vi "imp_test_v7.vi"() -> ()   [LabVIEW 2014]
uses:
  <vilib>/LabVIEW Targets/FPGA/cRIO/shared/nicrio_ModuleControls/nicrio_cRIO-9237_DataRatesRing.ctl
  <vilib>/LabVIEW Targets/FPGA/cRIO/shared/nicrio_ModuleControls/nicrio_cRIO-9237_ExcitationVoltageRing.ctl
  <vilib>/rvi/FXPMathLib/FxpSinAndCos/subVIs/nifxpmath_SinAndCos_SimConfig.ctl
  <vilib>/rvi/Emulation/niFpgaGetClockAttributes.vi
  <vilib>/rvi/Emulation/niFpgaSctlEmulationGetInTimedLoop.vi
  <vilib>/rvi/Emulation/niFpgaEmulationReportErrorSimple.vi
  <vilib>/rvi/Emulation/niFpgaProcessEmulError.vi
  <vilib>/rvi/interface/RandomDataEmulation/nirviRandomDataMultiElementFPGAFIFO.vi
  <instcachedir>/0/nirviRandomDataMultiElementFPGAFIFO_AD0CFC12EF974623A9C2E4184BC062B2.lvgen/nirviRandomDataMultiElementFPGAFIFO_AD0CFC12EF974623A9C2E4184BC062B2_025.vi
  <vilib>/rvi/interface/RandomDataEmulation/niFpgaRandomDataHandleErrors.vi
  <vilib>/rvi/Emulation/niFpgaCriticalErrorInLSC.vi
  <vilib>/rvi/eio/common/nirviEmuTemplateMethod_errors.vi
  <vilib>/rvi/FXPMathLib/FxpSinAndCos/simVIs/DllFxpSinAndCosTemp_sub.vi
  <vilib>/rvi/eio/common/nirviEmuTemplatePropertySet_errors.vi
  <vilib>/rvi/DataTransferAndStorage/Container/XNode/niFpgaContainer.xnode
  <vilib>/rvi/interface/RandomDataEmulation/nirviRandomDataFpgaMultiElementTemplate.vi
  <vilib>/eio/EIONode/EIONode.xnode
  <vilib>/rvi/FXPMathLib/FxpMul/XNode/nifxpmath_Multiplier.xnode
  <vilib>/rvi/FXPMathLib/FxpSinAndCos/XNode/nifxpmath_SinAndCos.xnode
  <vilib>/rvi/Analysis/measure/butterworth/XNode/niFpgaButterworthFilter.xnode
  <vilib>/rvi/FXPMathLib/FxpSub/XNode/nifxpmath_Sub.xnode
  <vilib>/rvi/FXPMathLib/FxpAdd/XNode/nifxpmath_Add.xnode
  <vilib>/eio/EIOPropertyNode/EIOPropertyNode.xnode
  <vilib>/rvi/eio/common/nirviEmuTemplatePropertyGet_errors.vi
  <vilib>/rvi/eio/common/nirviEmuTemplatePropertyGet_noerrors.vi
  <vilib>/rvi/eio/common/nirviEmuTemplatePropertySet_noerrors.vi
  <vilib>/rvi/FXPMathLib/sim/FxpSim.dll
panel:
  in  "Belt_op":fxp<+/-,7,7>
  in  "Belt_mp":fxp<+/-,6,6>
  in  "Belt_oy":fxp<+/-,7,7>
  in  "Belt_my":fxp<+/-,6,6>
  out "Fp_dc":fxp<+/-,32,10>
  out "Fy_dc":fxp<+/-,32,10>
  in  "Zero_y":bool
  in  "Zero_p":bool
  in  "mt0_omega_p":u32
  in  "Encoder reset":bool
  out "fpt_d":fxp<+/-,36,18>
  out "Dp_error_dd":fxp<+/-,36,16>
  out "Dp_error_d":fxp<+/-,33,8>
  in  "Dp_dd coeff.":i32[](array[numeric])=[946630756, 63555534]
  out "Dp_dd":fxp<+/-,36,25>
  out "dFp_PID":fxp<+/-,36,18>
  in  "dFp_PID coeff.":i32[](array[numeric])=[946630756, 63555534]
  out "fpt_i":fxp<+/-,34,18>
  in  "Bv_p":fxp<+/-,22,8>
  in  "Kv_p":fxp<+/-,22,8>
  out "Dp_error":fxp<+/-,22,7>
  out "Dpr_sin":fxp<+/-,22,7>
  in  "Sin offset_p":fxp<+/-,22,7>
  in  "Sin magnitude_p":fxp<+/-,21,6>
  out "Dpr_sin_dd":fxp<+/-,35,20>
  out "Dpr_sin_d":fxp<+/-,33,15>
  out "Sin omega_p":fxp<+/-,34,9>
  in  "Sin wave freq._p (Hz)":fxp<+/-,32,6>
  in  "Dpr_step":fxp<+/-,22,7>
  out "Dpr_for":fxp<+/-,22,7>
  in  "Command_p":i16(ring) items=["Step", "Sine"]
  in  "Ki_p":fxp<+/-,36,9>
  out "Fp_PID":fxp<+/-,36,16>
  in  "fp_tolorance":fxp<+,22,6>
  out "fp_tilde":fxp<+/-,33,10>
  in  "Kd_p":fxp<+/-,36,9>
  in  "Kp_p":fxp<+/-,36,9>
  out "Fr_p":fxp<+/-,32,10>
  in  "S/F coeff_p":fxp<+/-,25,-10>
  in  "S/F coeff_y":fxp<+/-,25,-10>
  out "va_p":fxp<+/-,36,7>
  out "vb_p":fxp<+/-,37,8>
  out "vq_p_F":fxp<+/-,20,5> format="%.57g"
  out "vd_p_F":fxp<+/-,20,5>
  in  "dFp_add":bool
  in  "Stop motor_p":bool
  out "Force_p":fxp<+/-,32,10>
  in  "Strain selection_p":i16(ring) items=["Raw", "Avg.8", "Avg.8 w. filter"]
  out "Strain_p (Avg8 w. f)":fxp<+/-,36,8>
  in  "Strain_p Avg.8 coeff.":i32[](array[numeric])=[946630756, 63555534]
  out "Strain_p (Avg8)":fxp<+/-,36,4>
  out "Raw Strain_p":fxp<+/-,36,4>
  out "Mod6/AI3":fxp<+/-,36,4>
  in  "Strain gage reset_p":bool
  out "Dp_d (mm/s)":fxp<+/-,36,11>
  out "omega_p (rad/s)":fxp<+/-,20,9>
  out "mt_omega_p":u32
  out "rad_p(NrTheta)":fxp<+/-,33,20>
  out "D_p(mm)":fxp<+/-,32,7>
  out "Encoder Position_p":i32
  in  "Encoder reset_p":bool
  out "Strain_y (Avg8 w. f)":fxp<+/-,36,8>
  in  "Strain_y Avg8 coeff.":i32[](array[numeric])=[-898916953, 1957103773, 3888751]
  out "Dyr_for":fxp<+/-,22,7>
  in  "Command_y":i16(ring) items=["Step", "Sine"]
  out "Strain_y (Avg8)":fxp<+/-,36,4>
  in  "Strain selection_y":i16(ring) items=["Raw", "Avg.8", "Avg.8 w. filter"]
  out "vb_y":fxp<+/-,38,8>
  out "va_y":fxp<+/-,38,8>
  out "fyt_d":fxp<+/-,36,18>
  out "Fr_y":fxp<+/-,32,10>
  in  "Bv_y":fxp<+/-,22,8>
  out "Dy_error_dd":fxp<+/-,36,16>
  out "Dy_error_d":fxp<+/-,33,8>
  in  "Kv_y":fxp<+/-,22,8>
  out "Dy_error":fxp<+/-,22,7>
  out "Dyr_sin_dd":fxp<+/-,35,20>
  out "Dyr_sin_d":fxp<+/-,33,15>
  out "Sin omega_y":fxp<+/-,34,9>
  out "Dyr_sin":fxp<+/-,22,7>
  in  "Sin offset_y":fxp<+/-,22,7>
  in  "Sin magnitude_y":fxp<+/-,21,6>
  out "Time now(s)":fxp<+,52,14>
  in  "Sin wave freq._y (Hz)":fxp<+/-,32,6>
  in  "Dyr_step":fxp<+/-,22,7>
  in  "Drive mode":i16(ring) items=["Backward", "Forward"]
  out "Dy_dd":fxp<+/-,36,25>
  in  "Dy_dd coeff.":i32[](array[numeric])=[946630756, 63555534]
  out "dFy_PID":fxp<+/-,36,18>
  in  "dFy_PID coeff.":i32[](array[numeric])=[946630756, 63555534]
  out "fyt_i":fxp<+/-,36,16>
  out "Fy_PID":fxp<+/-,36,16>
  in  "fy_tolorance":fxp<+,22,6>
  in  "Ki_y":fxp<+/-,36,9>
  in  "Kd_y":fxp<+/-,36,9>
  out "fy_tilde":fxp<+/-,32,10>
  in  "Kp_y":fxp<+/-,36,9>
  out "vq_y_F":fxp<+/-,20,5> format="%.57g"
  out "vd_y_F":fxp<+/-,20,5>
  in  "dFy_add":bool
  in  "Stop motor_y":bool
  out "Dy_d (mm/s)":fxp<+/-,36,11>
  out "omega_y (rad/s)":fxp<+/-,20,9>
  in  "mt0_omega_y":u32
  out "mt_omega_y":u32
  out "rad_y(NrTheta)":fxp<+/-,33,20>
  out "D_y(mm)":fxp<+/-,32,7>
  out "Encoder Position_y":i32
  in  "Encoder reset_y":bool
  in  "Ini coe.":bool
  out "Loop rate (kHz)":fxp<+/-,36,7>
  out "Force_y":fxp<+/-,32,10>
  out "Raw Strain_y":fxp<+/-,36,4>
  in  "Strain gage reset_y":bool
  in  "Stop (Strain)":bool
  out "Mod6/AI2":fxp<+/-,36,4>
  in  "Excitation Voltage":T1 items=["2.5 Volts", "3.3 Volts", "5.0 Volts", "10.0 Volts", "External Excitation"]
  in  "Data Rate":T2=1 items=["50.000 kS/s (NI 9237)"=1, "25.000 kS/s (NI 9237)"=2, "16.667 kS/s (NI 9237)"=3, "12.500 kS/s (NI 9237)"=4, "10.000 kS/s (NI 9237)"=5, "8.333 kS/s (NI 9237)"=6, "7.143 kS/s (NI 9237)"=7, "6.250 kS/s (NI 9237)"=8, "5.556 kS/s (NI 9237)"=9, "5.000 kS/s (NI 9237)"=10, "4.545 kS/s (NI 9237)"=11, "4.167 kS/s (NI 9237)"=12, "3.846 kS/s (NI 9237)"=13, "3.571 kS/s (NI 9237)"=14, "3.333 kS/s (NI 9237)"=15, "3.125 kS/s (NI 9237)"=16, "2.941 kS/s (NI 9237)"=17, "2.778 kS/s (NI 9237)"=18, "2.632 kS/s (NI 9237)"=19, "2.500 kS/s (NI 9237)"=20, "2.381 kS/s (NI 9237)"=21, "2.273 kS/s (NI 9237)"=22, "2.174 kS/s (NI 9237)"=23, "2.083 kS/s (NI 9237)"=24, "2.000 kS/s (NI 9237)"=25, "1.923 kS/s (NI 9237)"=26, "1.852 kS/s (NI 9237)"=27, "1.786 kS/s (NI 9237)"=28, "1.724 kS/s (NI 9237)"=29, "1.667 kS/s (NI 9237)"=30, "1.613 kS/s (NI 9237)"=31]
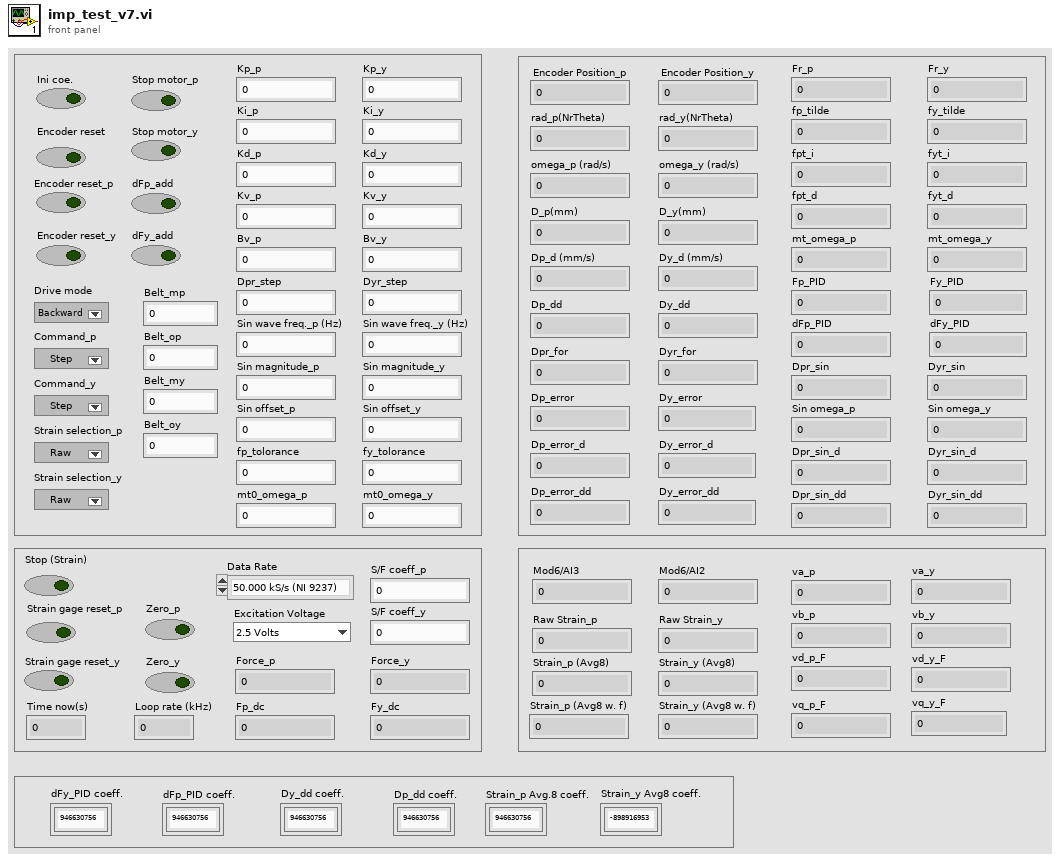
[diagram p1: front panel]
types:
  T1 = typedef "nicrio_cRIO-9237_ExcitationVoltageRing.ctl" = u8
  T2 = typedef "nicrio_cRIO-9237_DataRatesRing.ctl" = u8
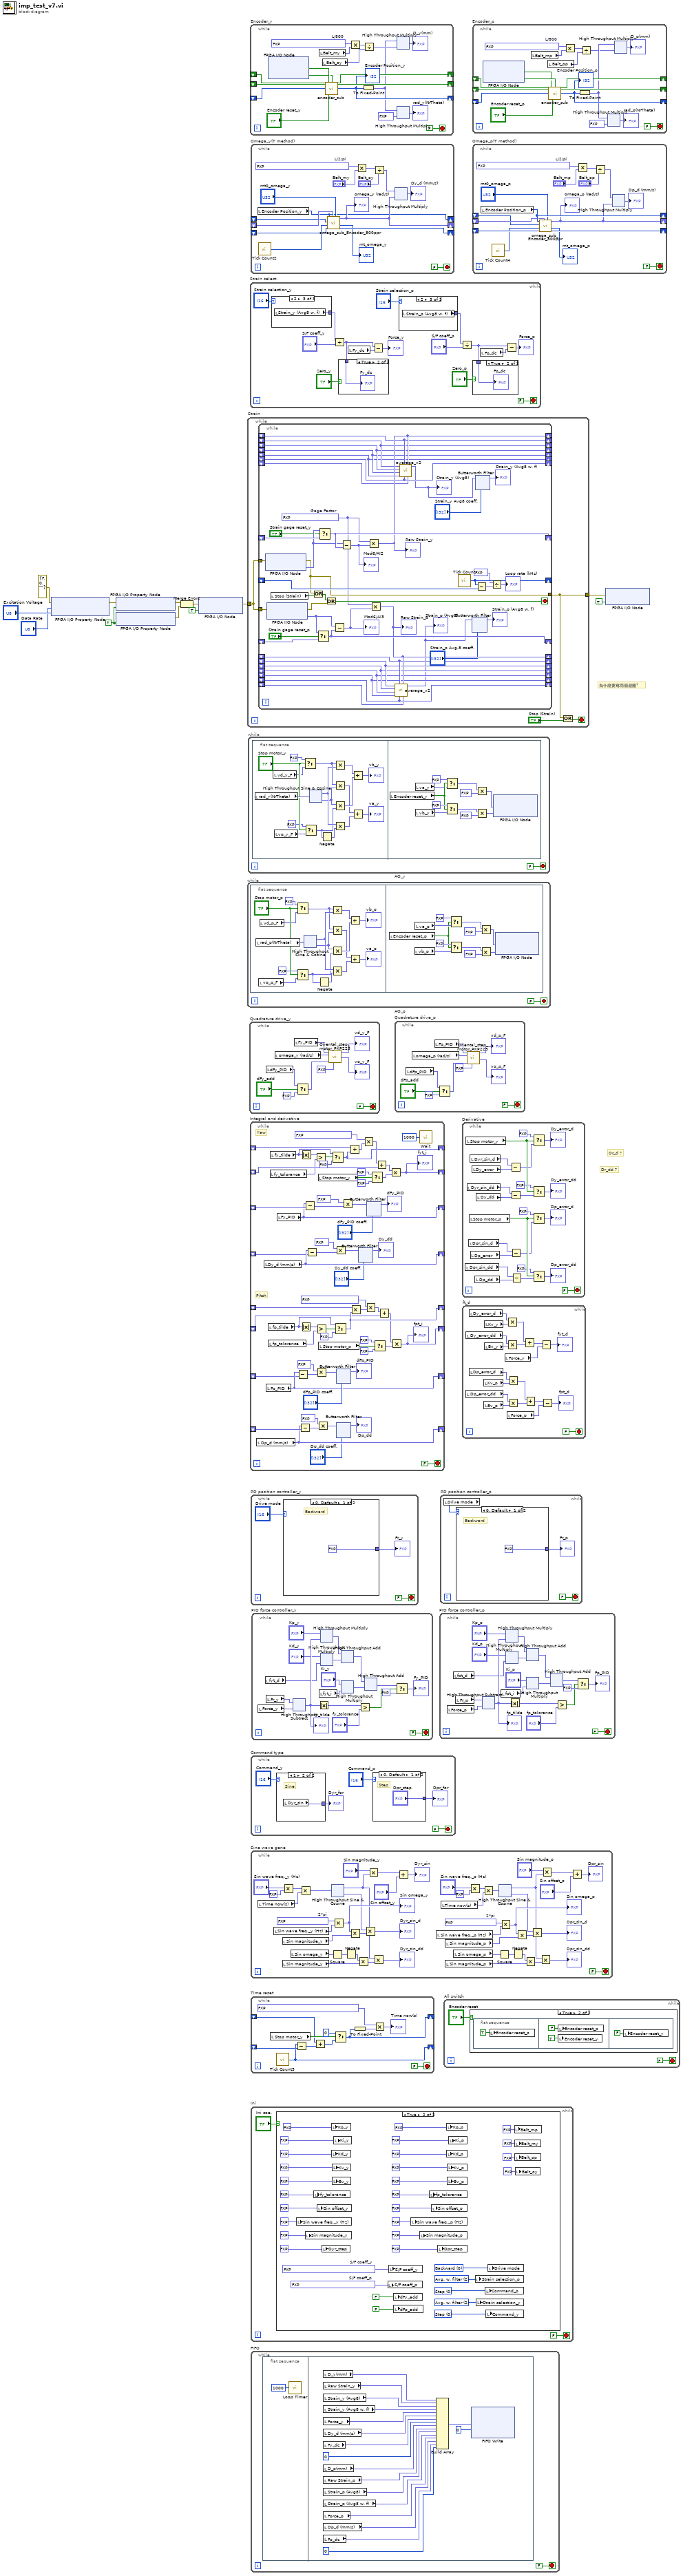
[diagram p0: block diagram]
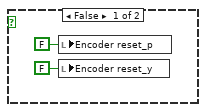
[diagram p2: hidden frame]
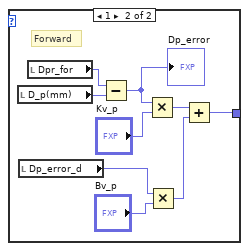
[diagram p3: hidden frame]
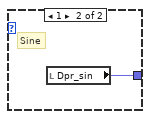
[diagram p4: hidden frame]
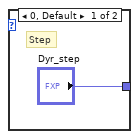
[diagram p5: hidden frame]
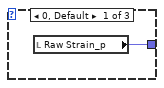
[diagram p8: hidden frame]
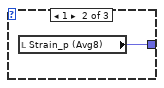
[diagram p9: hidden frame]
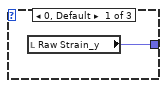
[diagram p10: hidden frame]
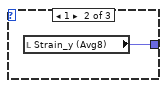
[diagram p11: hidden frame]
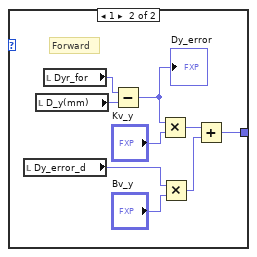
[diagram p12: hidden frame]
diagram:
  w5 = TRUE ("Half-Bridge Enable")
  # "為什麼要寫兩個迴圈?"
  # "Dr_dd ?"
  # "Dr_d ?"
  n1 = xnode "FPGA I/O Property Node"("error in"=errorcluster {"status"=FALSE, "code"=0, "source"=""}, "Data Rate"="Data Rate", "Excitation Voltage"="Excitation Voltage") -> ("error out"=w10:errorcluster)  [unwired: 1 in, 1 out]
  n2 = xnode "FPGA I/O Property Node"("error in"=w10, "Half-Bridge Enable"=w5) -> ("error out"=w3:errorcluster)  [unwired: 1 in, 1 out]
  n3 = xnode "FPGA I/O Property Node"("Half-Bridge Enable"=w5) -> ("error out"=w2:errorcluster)  [unwired: 2 in, 1 out]
  n4 = Merge Errors(w3, w2) -> (w4:errorcluster)
  n5 = xnode "FPGA I/O Node"("error in"=w4, "Mod6/Start"=TRUE) -> ("error out"=w8:errorcluster)  [unwired: 1 in, 1 out]
  n6 = while "Strain" {
    tunnel: w8 -> [w15]
    tunnel: [w13] -> w1
    stop <- w14 stop-if-true
    n7 = while {
      tunnel: w15 -> [w61]
      tunnel: [w34] -> w13
      shift-right: [w58] -> _
      shift-left: _ -> [w59]
      shift-right: [w54] -> _
      shift-left: _ -> [w55]
      shift-right: [w49] -> _
      shift-left: _ -> [w48]
      shift-right: [w48] -> _
      shift-left: _ -> [w47]
      shift-right: [w47] -> _
      shift-left: _ -> [w46]
      shift-right: [w46] -> _
      shift-left: _ -> [w45]
      shift-right: [w45] -> _
      shift-left: _ -> [w44]
      shift-right: [w44] -> _
      shift-left: _ -> [w43]
      shift-right: [w43] -> _
      shift-left: _ -> [w42]
      tunnel: w15 -> [w38]
      shift-right: [w31] -> _
      shift-left: _ -> [w32]
      shift-right: [w27] -> _
      shift-left: _ -> [w26]
      shift-right: [w26] -> _
      shift-left: _ -> [w25]
      shift-right: [w25] -> _
      shift-left: _ -> [w24]
      shift-right: [w24] -> _
      shift-left: _ -> [w23]
      shift-right: [w23] -> _
      shift-left: _ -> [w22]
      shift-right: [w22] -> _
      shift-left: _ -> [w21]
      shift-right: [w21] -> _
      shift-left: _ -> [w20]
      stop <- w35 stop-if-true
      w29 = fxp<+,20,2> 2.115001678466797  # Gage Factor
      n8 = xnode "FPGA I/O Node"("error in"=w61) -> ("error out"=w34:errorcluster, "Mod6/AI2"=w56:fxp<+/-,24,-4>)  [unwired: 1 in, 1 out]
      n9 = xnode "FPGA I/O Node"("error in"=w38) -> ("error out"=w36:errorcluster, "Mod6/AI3"=w30:fxp<+/-,24,-4>)  [unwired: 1 in, 1 out]
      n10 = local read "Stop (Strain)"() -> (w60:bool)
      n11 = Or(x=w34, y=w60) -> (x .or. y?=w37:bool)
      n12 = Select(t=w30, s="Strain gage reset_p", f=w32) -> (s? t:f=w31:fxp<+/-,24,-4>)
      n13 = Select(t=w56, s="Strain gage reset_y", f=w59) -> (s? t:f=w58:fxp<+/-,24,-4>)
      n14 = Or(x=w37, y=w36) -> (x .or. y?=w35:bool)
      n15 = Subtract(x=w30, y=w31) -> (x-y=w28:fxp<+/-,30,-3>)
      "Mod6/AI3" <- w28
      n16 = Subtract(x=w56, y=w58) -> (x-y=w57:fxp<+/-,30,-3>)
      "Mod6/AI2" <- w57
      n17 = Multiply(x=w29, y=w57) -> (x*y=w49:fxp<+/-,41,6>)
      "Raw Strain_y" <- w49
      n18 = Multiply(x=w29, y=w28) -> (x*y=w27:fxp<+/-,50,-1>)
      "Raw Strain_p" <- w27
      n19 = call "average_v2.vi"("Numeric 8"=w20, "Numeric"=w27, "Numeric 7"=w21, "Numeric 2"=w26, "Numeric 6"=w22, "Numeric 5"=w23, "Numeric 4"=w24, "Numeric 3"=w25) -> ("Mean (8pt)"=w19:fxp<+/-,32,4>)  [unwired: 1 in, 2 out]
      "Strain_p (Avg8)" <- w19
      n20 = call "average_v2.vi"("Numeric 8"=w42, "Numeric"=w49, "Numeric 7"=w43, "Numeric 2"=w48, "Numeric 6"=w44, "Numeric 5"=w45, "Numeric 4"=w46, "Numeric 3"=w47) -> ("Mean (8pt)"=w41:fxp<+/-,32,4>)  [unwired: 1 in, 2 out]
      "Strain_y (Avg8)" <- w41
      n21 = call "Tick Count"() -> ("Tick Count(uSec)"=w54:u32)
      n22 = xnode "Butterworth Filter"("input data"=w19, "scaled coefficients"="Strain_p Avg.8 coeff.") -> ("output data"=→"Strain_p (Avg8 w. f)":fxp<+/-,36,8>)  [unwired: 1 in]
      n23 = xnode "Butterworth Filter"("input data"=w41, "scaled coefficients"="Strain_y Avg8 coeff.") -> ("output data"=→"Strain_y (Avg8 w. f)":fxp<+/-,32,4>)  [unwired: 1 in]
      n24 = Subtract(x=w54, y=w55) -> (x-y=w52:fxp<+/-,32,16>)
      n25 = Divide(x=fxp<+,7,10> 1000.0, y=w52) -> (x/y=→"Loop rate (kHz)":fxp<+/-,40,27>)
    }
    n26 = Or(x=w13, y="Stop (Strain)") -> (x .or. y?=w14:bool)
  }
  n27 = while "AO_p" {
    stop <- FALSE stop-if-true
    n28 = flat-sequence {
      frame #0 {
        n29 = local read "rad_p(NrTheta)"() -> (w90:fxp<+/-,33,20>)
        n30 = local read "vq_p_F"() -> (w91:fxp<+/-,20,5>)
        n31 = local read "vd_p_F"() -> (w93:fxp<+/-,20,5>)
        n32 = Select(t=fxp<+/-,20,5> 0.0, s="Stop motor_p", f=w93) -> (s? t:f=w82:fxp<+/-,20,5>)
        n33 = Select(t=fxp<+,1,1> 0.0, s="Stop motor_p", f=w91) -> (s? t:f=w81:fxp<+/-,20,5>)
        n34 = xnode "High Throughput Sine & Cosine"("x (pi)"=w90) -> ("sin(x)"=w84:fxp<+/-,16,2>, "cos(x)"=w83:fxp<+/-,16,2>)
        n35 = Negate(x=w81) -> (-x=w89:fxp<+/-,21,6>)
        n36 = Multiply(x=w82, y=w84) -> (x*y=w88:fxp<+/-,36,7>)
        n37 = Multiply(x=w82, y=w83) -> (x*y=w86:fxp<+/-,36,7>)
        n38 = Multiply(x=w83, y=w81) -> (x*y=w87:fxp<+/-,36,7>)
        n39 = Multiply(x=w84, y=w89) -> (x*y=w85:fxp<+/-,35,6>)
        n40 = Add(x=w88, y=w87) -> (x+y=→"vb_p":fxp<+/-,37,8>)
        n41 = Add(x=w86, y=w85) -> (x+y=→"va_p":fxp<+/-,36,7>)
      }
      frame #1 {
        n42 = local read "Encoder reset_p"() -> (w126:bool)
        n43 = local read "vb_p"() -> (w127:fxp<+/-,37,8>)
        n44 = local read "va_p"() -> (w128:fxp<+/-,36,7>)
        n45 = Select(t=fxp<+,2,2> 3.0, s=w126, f=w128) -> (s? t:f=w134:fxp<+/-,36,7>)
        n46 = Select(t=fxp<+,1,1> 0.0, s=w126, f=w127) -> (s? t:f=w133:fxp<+/-,37,8>)
        n47 = Multiply(x=w134, y=fxp<+/-,1,0> -0.5) -> (x*y=w129:fxp<+/-,36,6>)
        n48 = Multiply(x=w133, y=fxp<+/-,1,0> -0.5) -> (x*y=w130:fxp<+/-,36,6>)
        n49 = xnode "FPGA I/O Node"("Mod8/AO0"=w129, "Mod8/AO1"=w130) -> ()  [unwired: 2 in, 2 out]
      }
    }
  }
  n50 = while "AO_y" {
    stop <- FALSE stop-if-true
    n51 = flat-sequence {
      frame #0 {
        n52 = local read "rad_y(NrTheta)"() -> (w154:fxp<+/-,33,20>)
        n53 = local read "vd_y_F"() -> (w152:fxp<+/-,20,5>)
        n54 = local read "vq_y_F"() -> (w151:fxp<+/-,20,5>)
        n55 = Select(t=fxp<+/-,20,5> 0.0, s="Stop motor_y", f=w152) -> (s? t:f=w146:fxp<+/-,20,5>)
        n56 = Select(t=fxp<+/-,20,5> 0.0, s="Stop motor_y", f=w151) -> (s? t:f=w145:fxp<+/-,20,5>)
        n57 = xnode "High Throughput Sine & Cosine"("x (pi)"=w154) -> ("sin(x)"=w148:fxp<+/-,17,2>, "cos(x)"=w147:fxp<+/-,17,2>)
        n58 = Negate(x=w145) -> (-x=w144:fxp<+/-,21,6>)
        n59 = Multiply(x=w146, y=w148) -> (x*y=w143:fxp<+/-,37,7>)
        n60 = Multiply(x=w146, y=w147) -> (x*y=w141:fxp<+/-,37,7>)
        n61 = Multiply(x=w147, y=w145) -> (x*y=w142:fxp<+/-,37,7>)
        n62 = Multiply(x=w148, y=w144) -> (x*y=w140:fxp<+/-,36,6>)
        n63 = Add(x=w143, y=w142) -> (x+y=→"vb_y":fxp<+/-,38,8>)
        n64 = Add(x=w141, y=w140) -> (x+y=→"va_y":fxp<+/-,37,7>)
      }
      frame #1 {
        n65 = local read "Encoder reset_y"() -> (w187:bool)
        n66 = local read "va_y"() -> (w186:fxp<+/-,38,8>)
        n67 = local read "vb_y"() -> (w185:fxp<+/-,38,8>)
        n68 = Select(t=fxp<+,2,2> 3.0, s=w187, f=w186) -> (s? t:f=w191:fxp<+/-,38,8>)
        n69 = Select(t=fxp<+,1,1> 0.0, s=w187, f=w185) -> (s? t:f=w190:fxp<+/-,38,8>)
        n70 = Multiply(x=w191, y=fxp<+/-,1,0> -0.5) -> (x*y=w194:fxp<+/-,39,8>)
        n71 = Multiply(x=w190, y=fxp<+/-,1,0> -0.5) -> (x*y=w195:fxp<+/-,37,6>)
        n72 = xnode "FPGA I/O Node"("Mod8/AO2"=w194, "Mod8/AO3"=w195) -> ()  [unwired: 2 in, 2 out]
      }
    }
  }
  n73 = while "Quadrature drive_y" {
    stop <- FALSE stop-if-true
    n74 = local read "dFy_PID"() -> (w197:fxp<+/-,36,18>)
    n75 = local read "omega_y (rad/s)"() -> (w205:fxp<+/-,20,9>)
    n76 = local read "Fy_PID"() -> (w198:fxp<+/-,36,16>)
    n77 = Select(t=w197, s="dFy_add", f=fxp<+,1,1> 0.0) -> (s? t:f=w201:fxp<+/-,36,18>)
    n78 = call "Oriental_step_motor_PKP225.vi"("F_Threshold"=fxp<+,12,12> 10.0, "dFmr"=w201, "omega"=w205, "Fmr"=w198) -> ("vq_F"=→"vq_y_F":fxp<+/-,20,5>, "vd_F"=→"vd_y_F":fxp<+/-,20,5>)  [unwired: 6 in]
  }
  n79 = while "Strain select." {
    stop <- FALSE stop-if-true
    n80 = case shown="2" "Strain selection_y" {
      tunnel: [w226 w227 w228] -> w219
      frame 0, Default {
        n81 = local read "Raw Strain_y"() -> (w226:fxp<+/-,36,4>)
      }
      frame 1 {
        n82 = local read "Strain_y (Avg8)"() -> (w227:fxp<+/-,36,4>)
      }
      frame 2 {
        n83 = local read "Strain_y (Avg8 w. f)"() -> (w228:fxp<+/-,36,8>)
      }
    }
    n84 = Divide(x=w219, y="S/F coeff_y") -> (x/y=w212:fxp<+/-,32,10>)
    n85 = case shown="True" "Zero_y" {
      tunnel: w212 -> [_ w222]
      frame False {
      }
      frame True {
        "Fy_dc" <- w222
      }
    }
    n86 = local read "Fy_dc"() -> (w213:fxp<+/-,32,10>)
    n87 = Subtract(x=w212, y=w213) -> (x-y=→"Force_y":fxp<+/-,33,11>)
    n88 = case shown="2" "Strain selection_p" {
      tunnel: [w223 w224 w225] -> w217
      frame 0, Default {
        n89 = local read "Raw Strain_p"() -> (w223:fxp<+/-,36,4>)
      }
      frame 1 {
        n90 = local read "Strain_p (Avg8)"() -> (w224:fxp<+/-,36,4>)
      }
      frame 2 {
        n91 = local read "Strain_p (Avg8 w. f)"() -> (w225:fxp<+/-,36,8>)
      }
    }
    n92 = Divide(x=w217, y="S/F coeff_p") -> (x/y=w209:fxp<+/-,32,10>)
    n93 = case shown="True" "Zero_p" {
      tunnel: w209 -> [_ w221]
      frame False {
      }
      frame True {
        "Fp_dc" <- w221
      }
    }
    n94 = local read "Fp_dc"() -> (w207:fxp<+/-,32,10>)
    n95 = Subtract(x=w209, y=w207) -> (x-y=→"Force_p":fxp<+/-,33,11>)
  }
  n96 = while "Integral and derivative" {
    shift-right: [w284] -> _
    shift-left: _ -> [w283]
    shift-right: [w276] -> _
    shift-left: _ -> [w275]
    shift-right: [w286] -> _
    shift-left: _ -> [w287]
    shift-right: [w266] -> _
    shift-left: _ -> [w265]
    shift-right: [w252] -> _
    shift-left: _ -> [w255]
    shift-right: [w245] -> _
    shift-left: _ -> [w244]
    shift-right: [w239] -> _
    shift-left: _ -> [w238]
    shift-right: [w234] -> _
    shift-left: _ -> [w235]
    stop <- FALSE stop-if-true
    # "Pitch"
    # "Yaw"
    n97 = local read "Dp_d (mm/s)"() -> (w234:fxp<+/-,36,11>)
    n98 = local read "Dy_d (mm/s)"() -> (w266:fxp<+/-,36,11>)
    n99 = local read "Fp_PID"() -> (w239:fxp<+/-,36,16>)
    n100 = local read "fp_tilde"() -> (w256:fxp<+/-,33,10>)
    n101 = local read "fp_tolorance"() -> (w259:fxp<+,22,6>)
    n102 = local read "fy_tolorance"() -> (w262:fxp<+,22,6>)
    n103 = local read "fy_tilde"() -> (w288:fxp<+/-,32,10>)
    n104 = local read "Fy_PID"() -> (w286:fxp<+/-,36,16>)
    n105 = Subtract(x=w239, y=w238) -> (x-y=w243:fxp<+/-,37,17>)
    n106 = Subtract(x=w234, y=w235) -> (x-y=w236:fxp<+/-,37,12>)
    n107 = Absolute Value(x=w256) -> (abs(x)=w260:fxp<+,33,10>)
    n108 = Absolute Value(x=w288) -> (abs(x)=w290:fxp<+,32,10>)
    n109 = Subtract(x=w286, y=w287) -> (x-y=w274:fxp<+/-,37,17>)
    n110 = Subtract(x=w266, y=w265) -> (x-y=w268:fxp<+/-,36,11>)
    n111 = Greater?(x=w290, y=w262) -> (0:w291:bool)
    n112 = Greater?(x=w260, y=w259) -> (0:w258:bool)
    n113 = Multiply(x=fxp<+,7,10> 1000.0, y=w243) -> (x*y=w241:fxp<+/-,32,18>)
    n114 = Multiply(x=fxp<+,7,10> 1000.0, y=w236) -> (x*y=w232:fxp<+/-,36,21>)
    n115 = local read "Stop motor_y"() -> (w277:bool)
    n116 = local read "Stop motor_p"() -> (w247:bool)
    n117 = Select(t=w288, s=w291, f=fxp<+/-,33,11> 0.0) -> (s? t:f=w284:fxp<+/-,33,11>)
    n118 = Select(t=w256, s=w258, f=fxp<+,1,1> 0.0) -> (s? t:f=w252:fxp<+/-,33,10>)
    n119 = Multiply(x=fxp<+,7,10> 1000.0, y=w268) -> (x*y=w267:fxp<+/-,36,21>)
    n120 = xnode "Butterworth Filter"("input data"=w241, "scaled coefficients"="dFp_PID coeff.") -> ("output data"=→"dFp_PID":fxp<+/-,36,22>)  [unwired: 1 in]
    n121 = xnode "Butterworth Filter"("input data"=w232, "scaled coefficients"="Dp_dd coeff.") -> ("output data"=→"Dp_dd":fxp<+/-,36,25>)  [unwired: 1 in]
    n122 = Multiply(x=fxp<+,7,10> 1000.0, y=w274) -> (x*y=w271:fxp<+/-,32,18>)
    n123 = Add(x=w283, y=w284) -> (x+y=w289:fxp<+/-,34,12>)
    n124 = Multiply(x=w255, y=w252) -> (x*y=w254:fxp<+/-,34,12>)
    n125 = xnode "Butterworth Filter"("input data"=w267, "scaled coefficients"="Dy_dd coeff.") -> ("output data"=→"Dy_dd":fxp<+/-,36,25>)  [unwired: 1 in]
    n126 = Multiply(x=fxp<+/-,30,12> 0.000499725341796875, y=w289) -> (x*y=w282:fxp<+/-,34,10>)
    n127 = Multiply(x=fxp<+/-,30,12> 0.000499725341796875, y=w254) -> (x*y=w251:fxp<+/-,34,10>)
    n128 = xnode "Butterworth Filter"("input data"=w271, "scaled coefficients"="dFy_PID coeff.") -> ("output data"=→"dFy_PID":fxp<+/-,36,22>)  [unwired: 1 in]
    n129 = Select(t=fxp<+,1,1> 0.0, s=w277, f=fxp<+,1,1> 1.0) -> (s? t:f=w280:fxp<+,1,1>)
    n130 = Select(t=fxp<+,1,1> 0.0, s=w247, f=fxp<+,1,1> 1.0) -> (s? t:f=w249:fxp<+,1,1>)
    n131 = Add(x=w282, y=w275) -> (x+y=w281:fxp<+/-,36,16>)
    n132 = Add(x=w251, y=w244) -> (x+y=w250:fxp<+/-,36,16>)
    n133 = Multiply(x=w281, y=w280) -> (x*y=w276:fxp<+/-,34,18>)
    "fyt_i" <- w276
    n134 = Multiply(x=w250, y=w249) -> (x*y=w245:fxp<+/-,34,18>)
    "fpt_i" <- w245
    n135 = call "Wait"("Count(uSec)"=u32 1000) -> ()  [unwired: 1 out]
  }
  n136 = while "Encoder_y" {
    shift-right: [w340] -> _
    shift-left: _ -> [w341]
    shift-right: [w342] -> _
    shift-left: _ -> [w343]
    shift-right: [w335] -> _
    shift-left: _ -> [w339]
    stop <- FALSE stop-if-true
    w329 = fxp<+/-,20,-5> 0.002499997615814209  # L/800
    n137 = xnode "FPGA I/O Node"() -> ("Mod4/DI3"=w338:bool, "Mod4/DI4"=w337:bool)  [unwired: 2 in, 2 out]
    n138 = local read "Belt_my"() -> (w328:fxp<+/-,6,6>)
    n139 = local read "Belt_oy"() -> (w326:fxp<+/-,7,7>)
    n140 = call "encoder_sub.vi"("A_pre"=w341, "B_pre"=w343, "Encoder Position_pre"=w339, "A input"=w338, "Encoder Position Reset"="Encoder reset_y", "B input"=w337) -> ("A"=w340:bool, "B"=w342:bool, "Encoder Position (Counts)"=w335:i32)  [unwired: 19 in]
    "Encoder Position_y" <- w335
    n141 = Multiply(x=w329, y=w328) -> (x*y=w327:fxp<+/-,26,1>)
    n142 = To Fixed-Point(number=w335) -> (fixed-point=w334:fxp<+/-,32,32>)  [unwired: 1 in]
    n143 = Divide(x=w327, y=w326) -> (x/y=w325:fxp<+/-,33,1>)
    n144 = xnode ("High Throughput Multiply")("x"=w334, "y"=w325) -> ("x*y"=→"D_y(mm)":fxp<+/-,64,33>)
    n145 = xnode ("High Throughput Multiply")("x"=w334, "y"=fxp<+/-,16,1> 0.125) -> ("x*y"=→"rad_y(NrTheta)":fxp<+/-,48,33>)
  }
  n146 = while "Omega_y(T method)" {
    shift-right: [w350] -> _
    shift-left: _ -> [w351]
    shift-right: [w353] -> _
    shift-left: _ -> [w355]
    shift-right: [w357] -> _
    shift-left: _ -> [w358]
    stop <- FALSE stop-if-true
    w348 = fxp<+/-,32,0> 0.3183098859153688  # L/2/pi
    n147 = local read "Encoder Position_y"() -> (w350:i32)
    n148 = call "Tick Count2"() -> ("Tick Count(Ticks)"=w359:u32)
    n149 = call "omega_sub_Encoder_800ppr.vi"("mt0"="mt0_omega_y", "omega_pre"=w355, "ticks_m_pre"=w358, "ticks"=w359, "count_pre"=w351, "count"=w350) -> ("ticks_m"=w357:u32, "mt"=→"mt_omega_y":u32, "omega"=w353:fxp<+/-,20,9>)  [unwired: 3 in]
    "omega_y (rad/s)" <- w353
    n150 = Multiply(x=w348, y="Belt_my") -> (x*y=w346:fxp<+/-,38,6>)
    n151 = Divide(x=w346, y="Belt_oy") -> (x/y=w344:fxp<+/-,20,1>)
    n152 = xnode ("High Throughput Multiply")("x"=w344, "y"=w353) -> ("x*y"=→"Dy_d (mm/s)":fxp<+/-,40,10>)
  }
  n153 = while "PD position controller_y" {
    stop <- FALSE stop-if-true
    n154 = case shown="0, Default" "Drive mode" {
      tunnel: [fxp<+/-,62,19> 0.0 w365] -> w361
      frame 0, Default {
        # "Backward"
      }
      frame 1 {
        # "Forward"
        n155 = local read "Dy_error_d"() -> (w367:fxp<+/-,33,8>)
        n156 = local read "D_y(mm)"() -> (w372:fxp<+/-,32,7>)
        n157 = local read "Dyr_for"() -> (w364:fxp<+/-,22,7>)
        n158 = Subtract(x=w364, y=w372) -> (x-y=w371:fxp<+/-,33,8>)
        "Dy_error" <- w371
        n159 = Multiply(x=w371, y="Kv_y") -> (x*y=w369:fxp<+/-,54,15>)
        n160 = Multiply(x=w367, y="Bv_y") -> (x*y=w366:fxp<+/-,55,16>)
        n161 = Add(x=w369, y=w366) -> (x+y=w365:fxp<+/-,55,16>)
      }
    }
    "Fr_y" <- w361
  }
  n162 = while "Command type" {
    stop <- FALSE stop-if-true
    n163 = case shown="1" "Command_y" {
      tunnel: ["Dyr_step" w381] -> w376
      frame 0, Default {
        # "Step"
      }
      frame 1 {
        # "Sine"
        n164 = local read "Dyr_sin"() -> (w381:fxp<+/-,22,7>)
      }
    }
    "Dyr_for" <- w376
    n165 = case shown="0, Default" "Command_p" {
      tunnel: ["Dpr_step" w379] -> w374
      frame 0, Default {
        # "Step"
      }
      frame 1 {
        # "Sine"
        n166 = local read "Dpr_sin"() -> (w379:fxp<+/-,22,7>)
      }
    }
    "Dpr_for" <- w374
  }
  n167 = while "Sine wave gene" {
    stop <- FALSE stop-if-true
    w387 = fxp<+,20,3> 6.2831878662109375  # 2*pi
    w419 = fxp<+,20,3> 6.2831878662109375  # 2*pi
    n168 = local read "Time now(s)"() -> (w425:fxp<+,52,14>)
    n169 = local read "Sin wave freq._y (Hz)"() -> (w418:fxp<+/-,32,6>)
    n170 = Multiply(x="Sin wave freq._y (Hz)", y=fxp<+/-,10,3> 2.0) -> (x*y=w426:fxp<+/-,41,9>)
    n171 = local read "Sin magnitude_y"() -> (w416:fxp<+/-,21,6>)
    n172 = local read "Sin magnitude_y"() -> (w409:fxp<+/-,21,6>)
    n173 = local read "Sin omega_y"() -> (w412:fxp<+/-,34,9>)
    n174 = Multiply(x=w426, y=w425) -> (x*y=w424:fxp<+/-,41,19>)
    n175 = Square(x=w412) -> (x^2=w411:fxp<+,34,18>)
    n176 = xnode "High Throughput Sine & Cosine"("x (pi)"=w424) -> ("sin(x)"=w406:fxp<+/-,16,2>, "cos(x)"=w414:fxp<+/-,16,2>)
    n177 = Multiply(x=w419, y=w418) -> (x*y=w417:fxp<+/-,34,9>)
    "Sin omega_y" <- w417
    n178 = Negate(x=w411) -> (-x=w410:fxp<+/-,35,19>)
    n179 = Multiply(x=w417, y=w416) -> (x*y=w415:fxp<+/-,33,15>)
    n180 = Multiply(x=w410, y=w409) -> (x*y=w408:fxp<+/-,34,20>)
    n181 = Multiply(x=w414, y=w415) -> (x*y=→"Dyr_sin_d":fxp<+/-,33,15>)
    n182 = Multiply(x="Sin magnitude_y", y=w406) -> (x*y=w422:fxp<+/-,37,8>)
    n183 = Multiply(x=w406, y=w408) -> (x*y=→"Dyr_sin_dd":fxp<+/-,35,20>)
    n184 = Add(x=w422, y="Sin offset_y") -> (x+y=→"Dyr_sin":fxp<+/-,37,8>)
    n185 = local read "Sin wave freq._p (Hz)"() -> (w383:fxp<+/-,32,6>)
    n186 = local read "Time now(s)"() -> (w401:fxp<+,52,14>)
    n187 = local read "Sin magnitude_p"() -> (w384:fxp<+/-,21,6>)
    n188 = local read "Sin magnitude_p"() -> (w386:fxp<+/-,21,6>)
    n189 = local read "Sin omega_p"() -> (w385:fxp<+/-,34,9>)
    n190 = Multiply(x="Sin wave freq._p (Hz)", y=fxp<+/-,10,3> 2.0) -> (x*y=w405:fxp<+/-,42,9>)
    n191 = Multiply(x=w405, y=w401) -> (x*y=w402:fxp<+/-,41,19>)
    n192 = Square(x=w385) -> (x^2=w397:fxp<+,34,18>)
    n193 = xnode "High Throughput Sine & Cosine"("x (pi)"=w402) -> ("sin(x)"=w388:fxp<+/-,16,2>, "cos(x)"=w393:fxp<+/-,16,2>)
    n194 = Multiply(x=w387, y=w383) -> (x*y=w400:fxp<+/-,34,9>)
    "Sin omega_p" <- w400
    n195 = Negate(x=w397) -> (-x=w396:fxp<+/-,35,19>)
    n196 = Multiply(x=w400, y=w384) -> (x*y=w399:fxp<+/-,33,15>)
    n197 = Multiply(x=w396, y=w386) -> (x*y=w395:fxp<+/-,35,19>)
    n198 = Multiply(x=w393, y=w399) -> (x*y=→"Dpr_sin_d":fxp<+/-,33,15>)
    n199 = Multiply(x=w388, y=w395) -> (x*y=→"Dpr_sin_dd":fxp<+/-,35,20>)
    n200 = Multiply(x="Sin magnitude_p", y=w388) -> (x*y=w391:fxp<+/-,37,8>)
    n201 = Add(x=w391, y="Sin offset_p") -> (x+y=→"Dpr_sin":fxp<+/-,37,8>)
  }
  n202 = while "Time reset" {
    shift-right: [w498] -> _
    shift-left: _ -> [w499]
    shift-right: [w493] -> _
    shift-left: _ -> [w494]
    stop <- FALSE stop-if-true
    n203 = local read "Stop motor_y"() -> (w500:bool)
    n204 = call "Tick Count3"() -> ("Tick Count(uSec)"=w498:u32)
    n205 = Subtract(x=w498, y=w499) -> (x-y=w497:u32)
    n206 = Add(x=w494, y=w497) -> (x+y=w496:u32)
    n207 = Select(t=u32 0, s=w500, f=w496) -> (s? t:f=w493:u32)
    n208 = To Fixed-Point(number=w493) -> (fixed-point=w492:fxp<+,32,32>)  [unwired: 1 in]
    n209 = Multiply(x=fxp<+,20,-18> 1.0000003385357559e-06, y=w492) -> (x*y=→"Time now(s)":fxp<+,52,14>)
  }
  n210 = while "Ini" {
    stop <- FALSE stop-if-true
    n211 = case shown="True" "Ini coe." {
      frame False {
      }
      frame True {
        w518 = i16 0 items=["Step", "Sine"] ("Command_p")
        w519 = i16 2 items=["Raw", "Avg.", "Avg. w. filter"] ("Strain selection_p")
        w520 = i16 0 items=["Step", "Sine"] ("Command_y")
        w521 = i16 2 items=["Raw", "Avg.", "Avg. w. filter"] ("Strain selection_y")
        w523 = fxp<+/-,25,-10> 5.851034075021744e-07  # S/F coeff_p
        w522 = fxp<+/-,25,-10> 1.0477961041033268e-06  # S/F coeff_y
        w529 = i16 0 items=["Backward", "Forward"] ("Drive mode")
        n212 = local write "Sin wave freq._y (Hz)"(fxp<+/-,32,6> 1.0 ("Sin wave freq. (Hz)")) -> ()
        n213 = local write "Sin magnitude_y"(fxp<+/-,22,7> 5.0 ("Sin magnitude")) -> ()
        n214 = local write "fy_tolorance"(fxp<+,22,6> 5.0 ("f_tolorance")) -> ()
        n215 = local write "Sin offset_y"(fxp<+/-,38,9> 0.0 ("Sin offset")) -> ()
        n216 = local write "Dyr_step"(fxp<+/-,22,7> 0.0 ("Dr")) -> ()
        n217 = local write "Kp_y"(fxp<+/-,36,9> 30.0 ("Kp")) -> ()
        n218 = local write "Kd_y"(fxp<+/-,36,9> 0.0 ("Kd")) -> ()
        n219 = local write "Kv_y"(fxp<+/-,22,8> 0.0 ("Kv")) -> ()
        n220 = local write "Bv_y"(fxp<+/-,22,8> 0.0 ("Bv")) -> ()
        n221 = local write "Ki_y"(fxp<+/-,36,9> 0.0 ("Ki")) -> ()
        n222 = local write "S/F coeff_p"(w523) -> ()
        n223 = local write "S/F coeff_y"(w522) -> ()
        n224 = local write "dFy_add"(FALSE ("dF_add")) -> ()
        n225 = local write "dFp_add"(FALSE ("dFp_add")) -> ()
        n226 = local write "Sin wave freq._p (Hz)"(fxp<+/-,32,6> 1.0 ("Sin wave freq._p (Hz)")) -> ()
        n227 = local write "Sin magnitude_p"(fxp<+/-,21,6> 5.0 ("Sin magnitude_p")) -> ()
        n228 = local write "fp_tolorance"(fxp<+,22,6> 5.0 ("fp_tolorance")) -> ()
        n229 = local write "Sin offset_p"(fxp<+/-,22,7> 0.0 ("Sin offset_p")) -> ()
        n230 = local write "Dpr_step"(fxp<+/-,22,7> 0.0 ("Dpr_step")) -> ()
        n231 = local write "Kp_p"(fxp<+/-,36,9> 30.0 ("Kp_p")) -> ()
        n232 = local write "Kd_p"(fxp<+/-,36,9> 0.0 ("Kd_p")) -> ()
        n233 = local write "Kv_p"(fxp<+/-,22,8> 0.0 ("Kv_p")) -> ()
        n234 = local write "Bv_p"(fxp<+/-,22,8> 0.0 ("Bv_p")) -> ()
        n235 = local write "Ki_p"(fxp<+/-,36,9> 0.0 ("Ki_p")) -> ()
        n236 = local write "Strain selection_p"(w519) -> ()
        n237 = local write "Strain selection_y"(w521) -> ()
        n238 = local write "Command_p"(w518) -> ()
        n239 = local write "Command_y"(w520) -> ()
        n240 = local write "Drive mode"(w529) -> ()
        n241 = local write "Belt_mp"(fxp<+/-,6,6> 16.0 ("Belt_mp")) -> ()
        n242 = local write "Belt_my"(fxp<+/-,6,6> 16.0 ("Belt_my")) -> ()
        n243 = local write "Belt_op"(fxp<+/-,7,7> 22.0 ("Belt_op")) -> ()
        n244 = local write "Belt_oy"(fxp<+/-,7,7> 22.0 ("Belt_oy")) -> ()
      }
    }
  }
  n245 = while "FIFO" {
    stop <- FALSE stop-if-true
    n246 = flat-sequence {
      frame #0 {
        n247 = call "Loop Timer"("Count(uSec)"=u32 1000) -> ()  [unwired: 1 out]
      }
      frame #1 {
        n248 = local read "D_y(mm)"() -> (w555:fxp<+/-,32,7>)
        n249 = local read "Raw Strain_y"() -> (w554:fxp<+/-,36,4>)
        n250 = local read "Strain_y (Avg8)"() -> (w553:fxp<+/-,36,4>)
        n251 = local read "Strain_y (Avg8 w. f)"() -> (w552:fxp<+/-,36,8>)
        n252 = local read "Force_y"() -> (w548:fxp<+/-,32,10>)
        n253 = local read "Dy_d (mm/s)"() -> (w549:fxp<+/-,36,11>)
        n254 = local read "Fy_dc"() -> (w550:fxp<+/-,32,10>)
        n255 = local read "D_p(mm)"() -> (w547:fxp<+/-,32,7>)
        n256 = local read "Raw Strain_p"() -> (w546:fxp<+/-,36,4>)
        n257 = local read "Strain_p (Avg8)"() -> (w545:fxp<+/-,36,4>)
        n258 = local read "Strain_p (Avg8 w. f)"() -> (w544:fxp<+/-,36,8>)
        n259 = local read "Force_p"() -> (w543:fxp<+/-,32,10>)
        n260 = local read "Dp_d (mm/s)"() -> (w542:fxp<+/-,36,11>)
        n261 = local read "Fp_dc"() -> (w541:fxp<+/-,32,10>)
        n262 = Build Array(w555, w554, w553, w552, w548, w549, w550, i16 0, w547, w546, w545, w544, w543, w542, w541, 0 ("element")) -> (w539:fxp<+/-,64,32>[])
        n263 = xnode ("FIFO Write")("Element"=w539, "Timeout"=0) -> ()  [unwired: 1 in, 2 out]
      }
    }
  }
  n264 = while "PID force controller_y" {
    stop <- FALSE stop-if-true
    n265 = local read "Force_y"() -> (w573:fxp<+/-,32,10>)
    n266 = local read "fyt_d"() -> (w557:fxp<+/-,36,18>)
    n267 = local read "Fr_y"() -> (w559:fxp<+/-,32,10>)
    n268 = xnode "High Throughput Subtract"("x"=w559, "y"=w573) -> ("x-y"=w572:fxp<+/-,33,11>)
    "fy_tilde" <- w572
    n269 = Absolute Value(x=w572) -> (abs(x)=w563:fxp<+,33,11>)
    n270 = local read "fyt_i"() -> (w558:fxp<+/-,36,16>)
    n271 = xnode ("High Throughput Multiply")("x"="Kp_y", "y"=w572) -> ("x*y"=w570:fxp<+/-,64,20>)
    n272 = xnode ("High Throughput Multiply")("x"="Kd_y", "y"=w557) -> ("x*y"=w569:fxp<+/-,64,27>)
    n273 = xnode ("High Throughput Add")("x"=w570, "y"=w569) -> ("x+y"=w566:fxp<+/-,64,28>)
    n274 = xnode ("High Throughput Multiply")("x"="Ki_y", "y"=w558) -> ("x*y"=w567:fxp<+/-,64,25>)
    n275 = Greater?(x=w563, y="fy_tolorance") -> (0:w561:bool)
    n276 = xnode ("High Throughput Add")("x"=w566, "y"=w567) -> ("x+y"=w565:fxp<+/-,64,29>)
    n277 = Select(t=w565, s=w561, f=fxp<+/-,51,14> 0.0) -> (s? t:f=→"Fy_PID":fxp<+/-,64,29>)
  }
  n278 = while "Quadrature drive_p" {
    stop <- FALSE stop-if-true
    n279 = local read "dFp_PID"() -> (w576:fxp<+/-,36,18>)
    n280 = local read "omega_p (rad/s)"() -> (w582:fxp<+/-,20,9>)
    n281 = local read "Fp_PID"() -> (w577:fxp<+/-,36,16>)
    n282 = Select(t=w576, s="dFp_add", f=fxp<+,1,1> 0.0) -> (s? t:f=w580:fxp<+/-,36,18>)
    n283 = call "Oriental_step_motor_PKP225.vi"("F_Threshold"=fxp<+,12,12> 10.0, "dFmr"=w580, "omega"=w582, "Fmr"=w577) -> ("vq_F"=→"vq_p_F":fxp<+/-,20,5>, "vd_F"=→"vd_p_F":fxp<+/-,20,5>)  [unwired: 6 in]
  }
  n284 = while "PID force controller_p" {
    stop <- FALSE stop-if-true
    n285 = local read "Force_p"() -> (w597:fxp<+/-,32,10>)
    n286 = local read "fpt_d"() -> (w588:fxp<+/-,36,18>)
    n287 = local read "Fr_p"() -> (w598:fxp<+/-,32,10>)
    n288 = xnode "High Throughput Subtract"("x"=w598, "y"=w597) -> ("x-y"=w589:fxp<+/-,33,11>)
    "fp_tilde" <- w589
    n289 = local read "fpt_i"() -> (w586:fxp<+/-,34,18>)
    n290 = xnode ("High Throughput Multiply")("x"="Kp_p", "y"=w589) -> ("x*y"=w587:fxp<+/-,64,20>)
    n291 = xnode ("High Throughput Multiply")("x"="Kd_p", "y"=w588) -> ("x*y"=w603:fxp<+/-,64,27>)
    n292 = Absolute Value(x=w589) -> (abs(x)=w596:fxp<+,33,11>)
    n293 = xnode ("High Throughput Add")("x"=w587, "y"=w603) -> ("x+y"=w601:fxp<+/-,64,28>)
    n294 = xnode ("High Throughput Multiply")("x"="Ki_p", "y"=w586) -> ("x*y"=w602:fxp<+/-,64,27>)
    n295 = xnode ("High Throughput Add")("x"=w601, "y"=w602) -> ("x+y"=w592:fxp<+/-,64,29>)
    n296 = Greater?(x=w596, y="fp_tolorance") -> (0:w593:bool)
    n297 = Select(t=w592, s=w593, f=fxp<+,1,1> 0.0) -> (s? t:f=→"Fp_PID":fxp<+/-,64,29>)
  }
  n298 = while "PD position controller_p" {
    stop <- FALSE stop-if-true
    n299 = local read "Drive mode"() -> (w606:i16)
    n300 = case shown="0, Default" w606 {
      tunnel: [fxp<+/-,62,19> 0.0 w609] -> w605
      frame 0, Default {
        # "Backward"
      }
      frame 1 {
        # "Forward"
        n301 = local read "D_p(mm)"() -> (w616:fxp<+/-,32,7>)
        n302 = local read "Dp_error_d"() -> (w608:fxp<+/-,33,8>)
        n303 = local read "Dpr_for"() -> (w615:fxp<+/-,22,7>)
        n304 = Subtract(x=w615, y=w616) -> (x-y=w614:fxp<+/-,24,8>)
        "Dp_error" <- w614
        n305 = Multiply(x=w614, y="Kv_p") -> (x*y=w611:fxp<+/-,34,16>)
        n306 = Multiply(x=w608, y="Bv_p") -> (x*y=w610:fxp<+/-,55,16>)
        n307 = Add(x=w611, y=w610) -> (x+y=w609:fxp<+/-,56,17>)
      }
    }
    "Fr_p" <- w605
  }
  n308 = while "All switch" {
    stop <- FALSE stop-if-true
    n309 = case shown="True" "Encoder reset" {
      frame False {
        n310 = local write "Encoder reset_p"(FALSE ("Encoder reset_p")) -> ()
        n311 = local write "Encoder reset_y"(FALSE ("Encoder reset_y")) -> ()
      }
      frame True {
        n312 = flat-sequence {
          frame #0 {
            n313 = local write "Encoder reset_p"(TRUE ("Encoder reset_p")) -> ()
          }
          frame #1 {
            n314 = local write "Encoder reset_y"(TRUE ("Encoder reset_y")) -> ()
            n315 = local write "Encoder reset_p"(FALSE ("Encoder reset_p")) -> ()
          }
          frame #2 {
            n316 = local write "Encoder reset_y"(FALSE ("Encoder reset_y")) -> ()
          }
        }
      }
    }
  }
  n317 = while "Derivative" {
    stop <- FALSE stop-if-true
    n318 = local read "Dpr_sin_dd"() -> (w633:fxp<+/-,35,20>)
    n319 = local read "Stop motor_y"() -> (w639:bool)
    n320 = local read "Dyr_sin_dd"() -> (w641:fxp<+/-,35,20>)
    n321 = local read "Dpr_sin_d"() -> (w635:fxp<+/-,33,15>)
    n322 = local read "Stop motor_p"() -> (w631:bool)
    n323 = local read "Dyr_sin_d"() -> (w644:fxp<+/-,33,15>)
    n324 = local read "Dp_error"() -> (w636:fxp<+/-,22,7>)
    n325 = local read "Dy_error"() -> (w645:fxp<+/-,22,7>)
    n326 = local read "Dp_dd"() -> (w634:fxp<+/-,36,25>)
    n327 = local read "Dy_dd"() -> (w642:fxp<+/-,36,25>)
    n328 = Subtract(x=w644, y=w645) -> (x-y=w643:fxp<+/-,34,16>)
    n329 = Subtract(x=w641, y=w642) -> (x-y=w640:fxp<+/-,41,26>)
    n330 = Subtract(x=w635, y=w636) -> (x-y=w628:fxp<+/-,34,16>)
    n331 = Subtract(x=w633, y=w634) -> (x-y=w632:fxp<+/-,41,26>)
    n332 = Select(t=fxp<+,1,1> 0.0, s=w639, f=w643) -> (s? t:f=→"Dy_error_d":fxp<+/-,34,16>)
    n333 = Select(t=fxp<+/-,64,49> 0.0, s=w639, f=w640) -> (s? t:f=→"Dy_error_dd":fxp<+/-,64,49>)
    n334 = Select(t=fxp<+,1,1> 0.0, s=w631, f=w628) -> (s? t:f=→"Dp_error_d":fxp<+/-,34,16>)
    n335 = Select(t=fxp<+/-,41,26> 0.0, s=w631, f=w632) -> (s? t:f=→"Dp_error_dd":fxp<+/-,41,26>)
  }
  n336 = while "ft_d" {
    stop <- FALSE stop-if-true
    n337 = local read "Dy_error_dd"() -> (w663:fxp<+/-,36,16>)
    n338 = local read "Dp_error_dd"() -> (w654:fxp<+/-,36,16>)
    n339 = local read "Dy_error_d"() -> (w665:fxp<+/-,33,8>)
    n340 = local read "Dp_error_d"() -> (w656:fxp<+/-,33,8>)
    n341 = local read "Kv_p"() -> (w657:fxp<+/-,22,8>)
    n342 = local read "Bv_p"() -> (w655:fxp<+/-,22,8>)
    n343 = local read "Kv_y"() -> (w666:fxp<+/-,22,8>)
    n344 = local read "Bv_y"() -> (w664:fxp<+/-,22,8>)
    n345 = local read "Force_y"() -> (w659:fxp<+/-,32,10>)
    n346 = Multiply(x=w665, y=w666) -> (x*y=w661:fxp<+/-,55,16>)
    n347 = Multiply(x=w663, y=w664) -> (x*y=w662:fxp<+/-,58,24>)
    n348 = Multiply(x=w656, y=w657) -> (x*y=w652:fxp<+/-,55,16>)
    n349 = Multiply(x=w654, y=w655) -> (x*y=w653:fxp<+/-,58,24>)
    n350 = local read "Force_p"() -> (w650:fxp<+/-,32,10>)
    n351 = Add(x=w661, y=w662) -> (x+y=w660:fxp<+/-,63,24>)
    n352 = Add(x=w652, y=w653) -> (x+y=w651:fxp<+/-,63,24>)
    n353 = Subtract(x=w660, y=w659) -> (x-y=→"fyt_d":fxp<+/-,63,24>)
    n354 = Subtract(x=w651, y=w650) -> (x-y=→"fpt_d":fxp<+/-,63,24>)
  }
  n355 = while "Encoder_p" {
    shift-right: [w681] -> _
    shift-left: _ -> [w682]
    shift-right: [w683] -> _
    shift-left: _ -> [w684]
    shift-right: [w677] -> _
    shift-left: _ -> [w685]
    stop <- FALSE stop-if-true
    w671 = fxp<+/-,20,-5> 0.002499997615814209  # L/800
    n356 = xnode "FPGA I/O Node"() -> ("Mod4/DI0"=w679:bool, "Mod4/DI1"=w680:bool)  [unwired: 2 in, 2 out]
    n357 = local read "Belt_mp"() -> (w670:fxp<+/-,6,6>)
    n358 = local read "Belt_op"() -> (w668:fxp<+/-,7,7>)
    n359 = call "encoder_sub.vi"("A_pre"=w682, "B_pre"=w684, "Encoder Position_pre"=w685, "A input"=w679, "Encoder Position Reset"="Encoder reset_p", "B input"=w680) -> ("A"=w681:bool, "B"=w683:bool, "Encoder Position (Counts)"=w677:i32)  [unwired: 19 in]
    "Encoder Position_p" <- w677
    n360 = Multiply(x=w671, y=w670) -> (x*y=w669:fxp<+/-,26,1>)
    n361 = To Fixed-Point(number=w677) -> (fixed-point=w676:fxp<+/-,32,32>)  [unwired: 1 in]
    n362 = Divide(x=w669, y=w668) -> (x/y=w667:fxp<+/-,33,1>)
    n363 = xnode ("High Throughput Multiply")("x"=w676, "y"=fxp<+/-,16,1> 0.125) -> ("x*y"=→"rad_p(NrTheta)":fxp<+/-,48,33>)
    n364 = xnode ("High Throughput Multiply")("x"=w676, "y"=w667) -> ("x*y"=→"D_p(mm)":fxp<+/-,64,33>)
  }
  n365 = while "Omega_p(T method)" {
    shift-right: [w701] -> _
    shift-left: _ -> [w699]
    shift-right: [w694] -> _
    shift-left: _ -> [w700]
    shift-right: [w696] -> _
    shift-left: _ -> [w698]
    stop <- FALSE stop-if-true
    w690 = fxp<+/-,32,0> 0.3183098859153688  # L/2/pi
    n366 = local read "Encoder Position_p"() -> (w701:i32)
    n367 = call "Tick Count4"() -> ("Tick Count(Ticks)"=w697:u32)
    n368 = call "omega_sub_Encoder_800ppr.vi"("mt0"="mt0_omega_p", "omega_pre"=w700, "ticks_m_pre"=w698, "ticks"=w697, "count_pre"=w699, "count"=w701) -> ("ticks_m"=w696:u32, "mt"=→"mt_omega_p":u32, "omega"=w694:fxp<+/-,20,9>)  [unwired: 3 in]
    "omega_p (rad/s)" <- w694
    n369 = Multiply(x=w690, y="Belt_mp") -> (x*y=w688:fxp<+/-,38,6>)
    n370 = Divide(x=w688, y="Belt_op") -> (x/y=w686:fxp<+/-,20,1>)
    n371 = xnode ("High Throughput Multiply")("x"=w686, "y"=w694) -> ("x*y"=→"Dp_d (mm/s)":fxp<+/-,40,10>)
  }
  n372 = xnode "FPGA I/O Node"("error in"=w1, "Mod6/Stop"=TRUE) -> ()  [unwired: 1 in, 2 out]
